vi "Owl429_TxAcyclicTransferConfig_isSdiEnabled.vi"(8 "error in (no error)":errorcluster, 11 "acyclic config handle":u32) -> (0 "error out":errorcluster, 2 "sdi enabled":bool, 3 "acyclic config handle":u32)   [LabVIEW 2015, in "AIT 429 System Explorer.lvlib"]
doc: "Indicates if SDI is enabled for the label transfer.\n\nReturns:\nTrue if SDI is enabled."
uses:
  AIT 429 System Explorer.lvlib
  <userlib>/ARINC-429/Owl429.lvlib
  owl429.dll
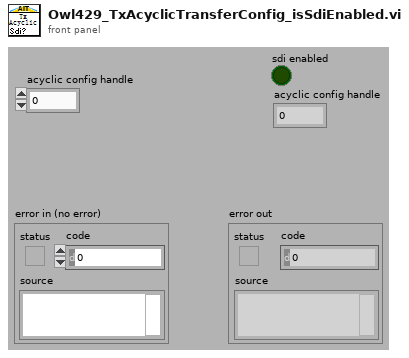
[diagram p1: front panel]
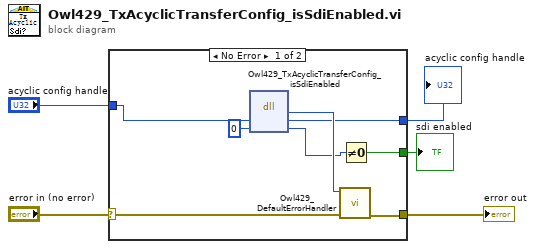
[diagram p0: block diagram]
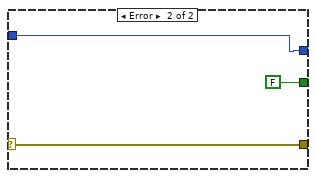
[diagram p2: hidden frame]
diagram:
  n1 = case shown="No Error" "error in (no error)" {
    selector: "error in (no error)" -> [w11 w16]
    tunnel: [w10 w16] -> w4
    tunnel: "acyclic config handle" -> [w12 w15]
    tunnel: [w8 FALSE] -> w2
    tunnel: [w7 w15] -> w1
    frame No Error {
      n2 = dll-call lib="owl429.*" fn="Owl429_TxAcyclicTransferConfig_isSdiEnabled" ("429owl.*:Owl429_TxScheduledLabelConfig_isSdiEnabled")("label config handle"=w12, "sdi enabled"=u8 0) -> ("return type"=w13:i32, "label config handle"=w7:u32, "sdi enabled"=w9:u8)  [unwired: 3 in, 2 out]
      n3 = call <userlib>:"Owl429_DefaultErrorHandler.vi"("error in (no error)"=w11, "error code"=w13) -> ("error out"=w10:errorcluster)  [unwired: 9 in]
      n4 = Not Equal To 0?(x=w9) -> (x != 0?=w8:bool)
    }
    frame Error {
    }
  }
  "error out" <- w4
  "sdi enabled" <- w2
  "acyclic config handle" <- w1
